vi "Init Error Handler.vi"(8 "error in":errorcluster, 11 "File Names (Optional)":string[](array[string])) -> (0 "error out":errorcluster)   [LabVIEW 2021]
doc: "Searches for a files named <b>*errors.xml</b> (default) in application directory and its subfolders. Optionally the file names can be specified at the input <b>File Names (Optional)</b>. \nThe XML file has to be in format of XML file which is generated by LabVIEW build-in Error Code Editor.\nError codes from the XML can be after the initialization used by using <b>Generate Error VI</b>."
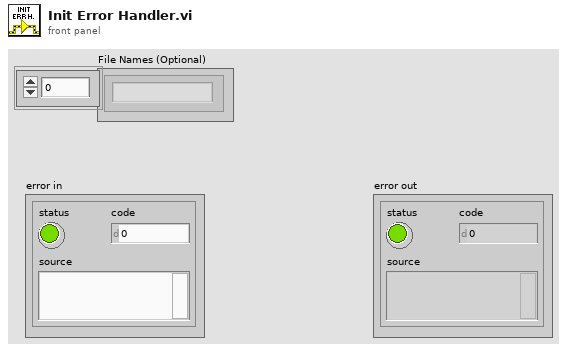
[diagram p1: front panel]
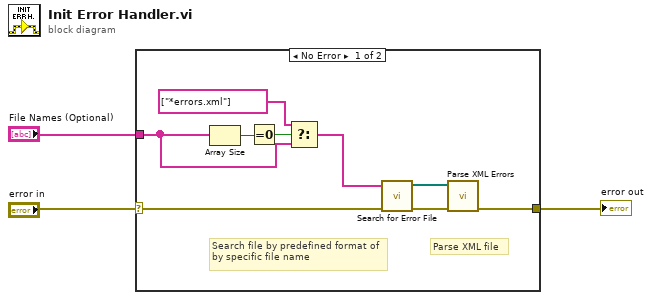
[diagram p0: block diagram]
diagram:
  n1 = case shown="No Error" "error in" {
    selector: "error in" -> [w9 w13]
    tunnel: [w10 w13] -> w3
    tunnel: "File Names (Optional)" -> [w6 _]
    frame No Error {
      # "Parse XML file"
      # "Search file by predefined format of by specific file name"
      n2 = Array Size(array=w6) -> (size(s)=w4:i32)
      n3 = Equal To 0?(x=w4) -> (x = 0?=w5:bool)
      n4 = Select(t=string[] ["*errors.xml"] ("string"), s=w5, f=w6) -> (s? t:f=w7:string[])
      n5 = call "Search for Error File.vi"("error in"=w9, "File Pattern"=w7) -> ("error out"=w12:errorcluster, "File Path"=w11:path[])  [unwired: 8 in]
      n6 = call "Parse XML Errors.vi"("error in"=w12, "XML File Path"=w11) -> ("error out"=w10:errorcluster)  [unwired: 9 in]
    }
    frame Error {
    }
  }
  "error out" <- w3
